vi "AFG Report Event.vi"(8 "error in (no error)":errorcluster, 9 "Event Data":variant, 10 "Report Events":T1=enum."Inited", 11 "I_AFG in":refnum<class "I_AFG.lvclass">) -> (0 "error out":errorcluster, 3 "I_AFG out":refnum<class "I_AFG.lvclass">)   [LabVIEW 2020, in "Actor_AFG.lvlib" / "I_AFG.lvclass"]
uses:
  I_AFG.lvclass
  AFG_Event.ctl
  Actor_AFG/Actor_AFG.lvclass
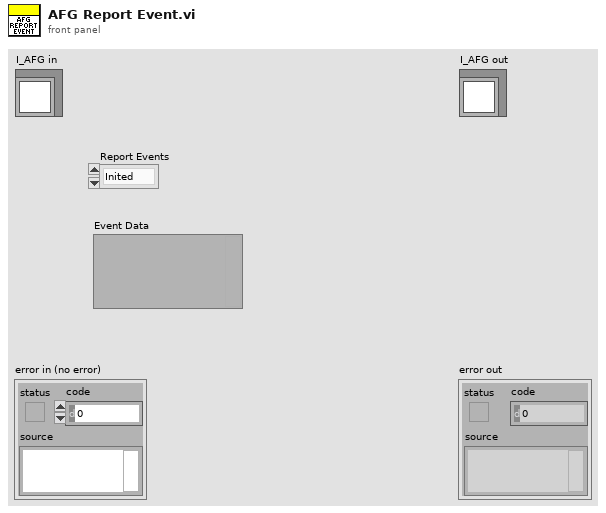
[diagram p1: front panel]
types:
  T1 = typedef "Actor_AFG.lvlib/Actor_AFG.lvclass/AFG_Event.ctl" = enum16{"General Event", "Inited", "Output", "Waveform Set", "Error"}
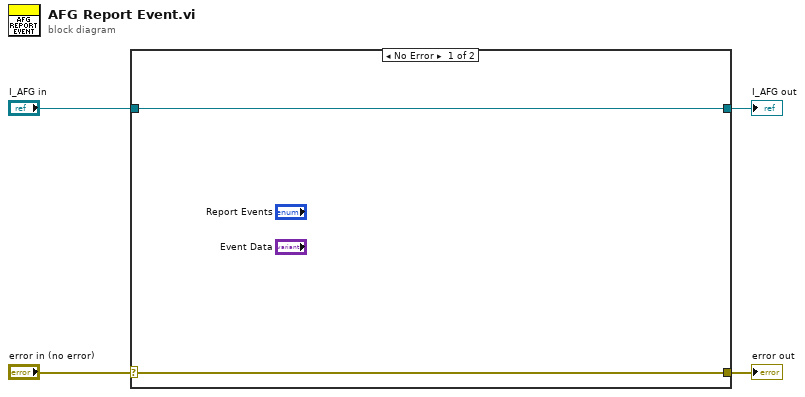
[diagram p0: block diagram]
diagram:
  n1 = case shown="No Error" "error in (no error)" {
    selector: "error in (no error)" -> [w5 w8]
    tunnel: [w5 w8] -> w3
    tunnel: [w6 w7] -> w1
    tunnel: "I_AFG in" -> [w6 w7]
    frame No Error {
    }
    frame Error {
    }
  }
  "error out" <- w3
  "I_AFG out" <- w1
